vi "Actor Core.vi"(8 "error in":errorcluster, 11 "Main in":refnum<class "Main.lvclass">) -> (0 "error out":errorcluster, 3 "Actor out":refnum<class "Actor.lvclass">)   [LabVIEW 2023, in "Main.lvlib" / "Main.lvclass"]
doc: "The user interface for this panel.\n\n----\nPlease see the following web address for additional documentation and tutorial information:\nhttp://www.mooregoodideas.com/mgi-panel-manager/\n\nAuthor: Derek Trepanier\n\nCopyright (c) 2018, Moore Good Ideas, Inc.\n\nAll rights reserved.\n\nRedistribution and use in source and binary forms, with or without modification, are permitted provided that the following conditions are met:\n\n * Redistributions of source code must retain the above copyright notice, this list of conditions and the following disclaimer.\n * Redistributions in binary form must reproduce the above copyright notice, this list of conditions and the following disclaimer in the documentation and/or other materials provided with the distribution.\n * Neither the name of Moore Good Ideas, Inc. nor the names of its contributors may be used to endorse or promote products derived from this software without specific prior written permission.\n\nTHIS SOFTWARE IS PROVIDED BY THE COPYRIGHT HOLDERS AND CONTRIBUTORS \"AS IS\" AND ANY EXPRESS OR IMPLIED WARRANTIES, INCLUDING, BUT NOT LIMITED TO, THE IMPLIED WARRANTIES OF MERCHANTABILITY AND FITNESS FOR A PARTICULAR PURPOSE ARE DISCLAIMED. IN NO EVENT SHALL THE COPYRIGHT OWNER OR CONTRIBUTORS BE LIABLE FOR ANY DIRECT, INDIRECT, INCIDENTAL, SPECIAL, EXEMPLARY, OR CONSEQUENTIAL DAMAGES (INCLUDING, BUT NOT LIMITED TO, PROCUREMENT OF SUBSTITUTE GOODS OR SERVICES; LOSS OF USE, DATA, OR PROFITS; OR BUSINESS INTERRUPTION) HOWEVER CAUSED AND ON ANY THEORY OF LIABILITY, WHETHER IN CONTRACT, STRICT LIABILITY, OR TORT (INCLUDING NEGLIGENCE OR OTHERWISE) ARISING IN ANY WAY OUT OF THE USE OF THIS SOFTWARE, EVEN IF ADVISED OF THE POSSIBILITY OF SUCH DAMAGE."
uses:
  Library/Main.lvclass
  builds/Framework/Actor Framework.lvlibp/1abvi3w/vi.lib/ActorFramework/Actor/Actor.lvclass
  Main Messages/Menu Response Msg/Menu Response Msg.lvclass/Menu Response Msg.ctl
  builds/Framework/Actor Framework.lvlibp/1abvi3w/vi.lib/ActorFramework/Message Enqueuer/Enqueue.vi
  Main Messages/Menu Response Msg/Menu Response Msg.lvclass
  builds/Framework/Engine.lvlibp/Managed Actor/Library/Managed Actor.lvclass
  builds/Framework/Engine.lvlibp/Engine/Library/Engine.lvclass
  builds/Framework/Actor Framework.lvlibp/1abvi3w/vi.lib/ActorFramework/Stop Msg/Stop Msg.lvclass
  C:/Users/Public/Documents/Development/builds/Framework/Engine.lvlibp/Engine/Library/Engine.lvclass
panel:
  in  "report":bool
  in  "configuration":bool
  in  "manual":bool
  in  "login":bool
  in  "uutinfo":bool
  out "Up Time:":string
  out "Serial:":string
  out "Model:":string
  out "Witness:":string
  out "Operator:":string
  out "Status":string
  out "Version":string caption="v"
  out "MissionLogo":picture
  out "CompanyLogo":picture
  out "Time":timestamp format="%<%I:%M:%S %p\n%x>T"
  in  "E-Stop":bool
  out "SplashScreen":picture
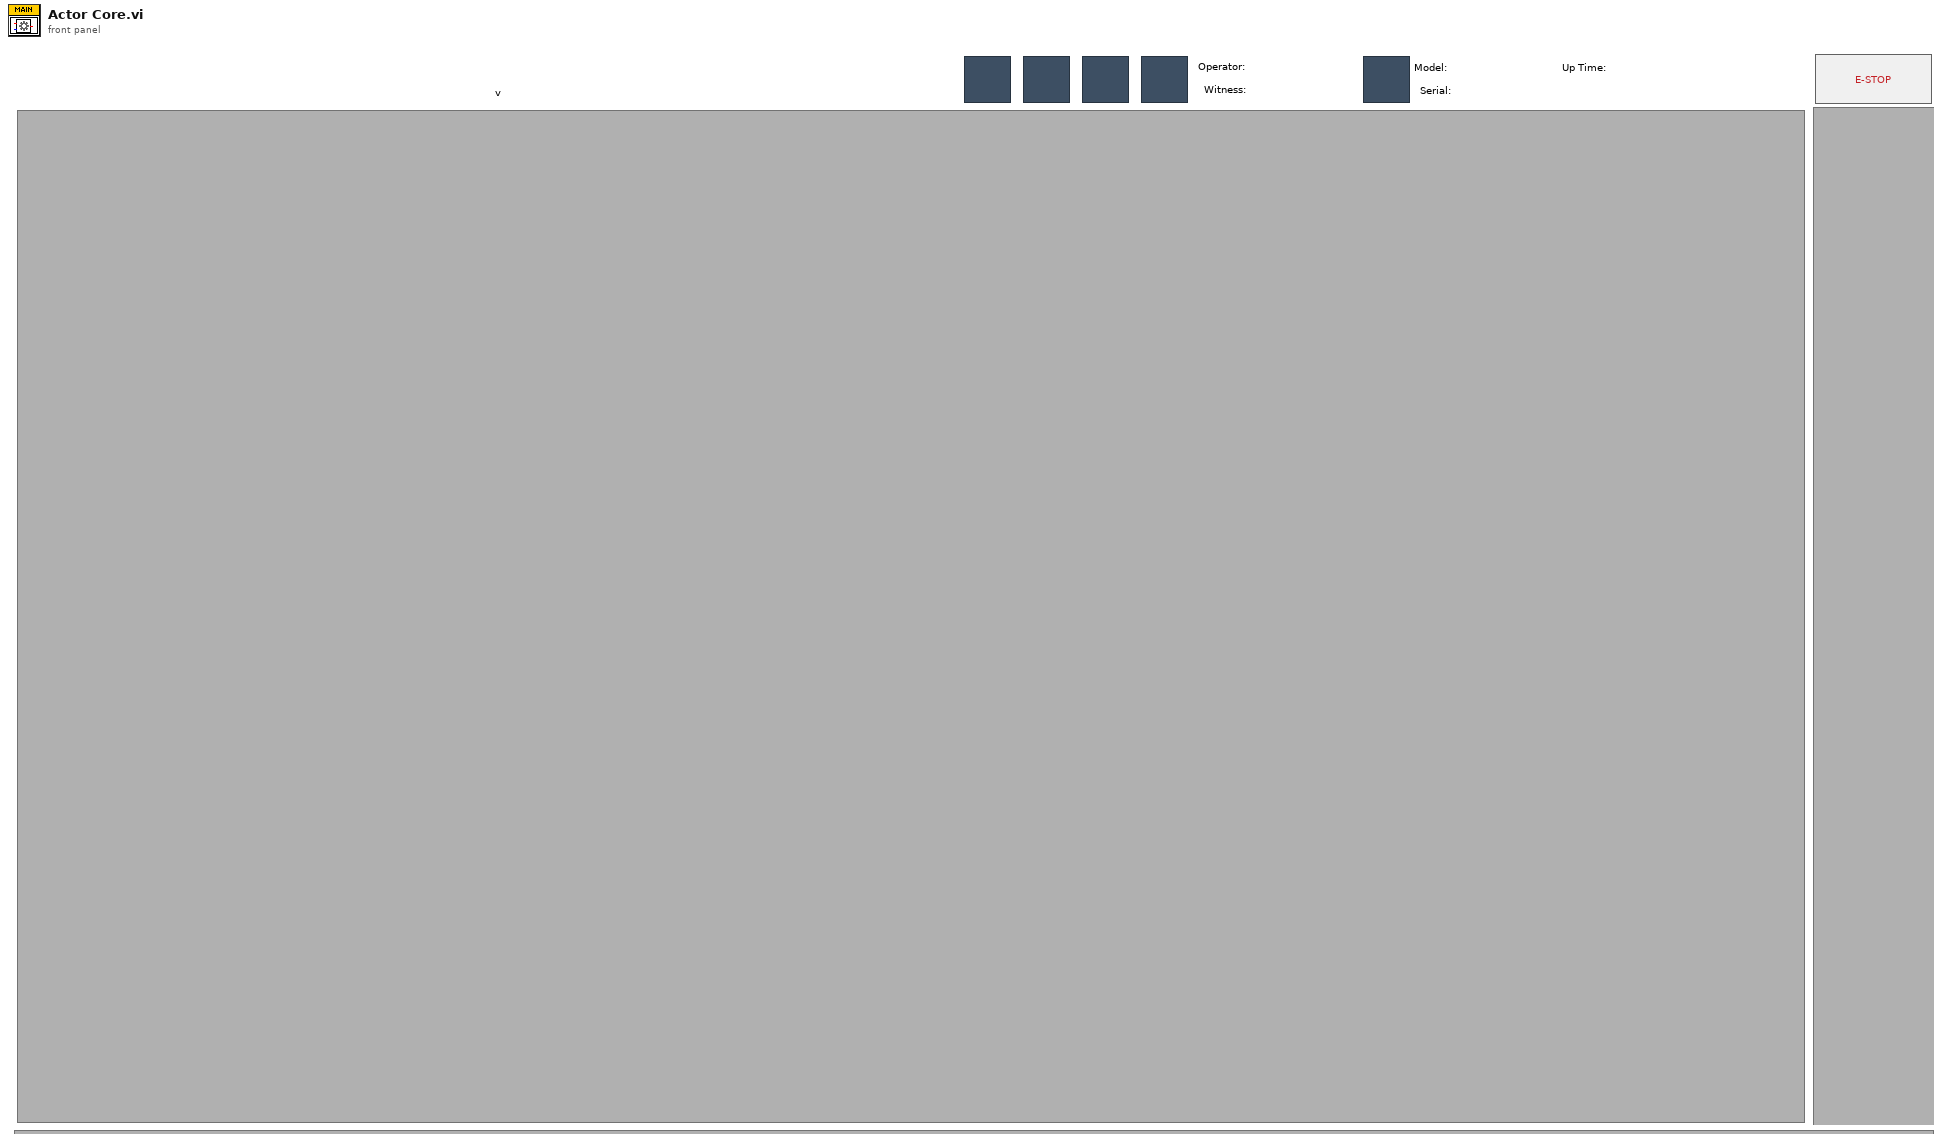
[diagram p1: front panel]
types:
  T1 = cluster{"Pnl Actor":refnum<event-registration>, "Event Registration Refnum":refnum<event-registration>}
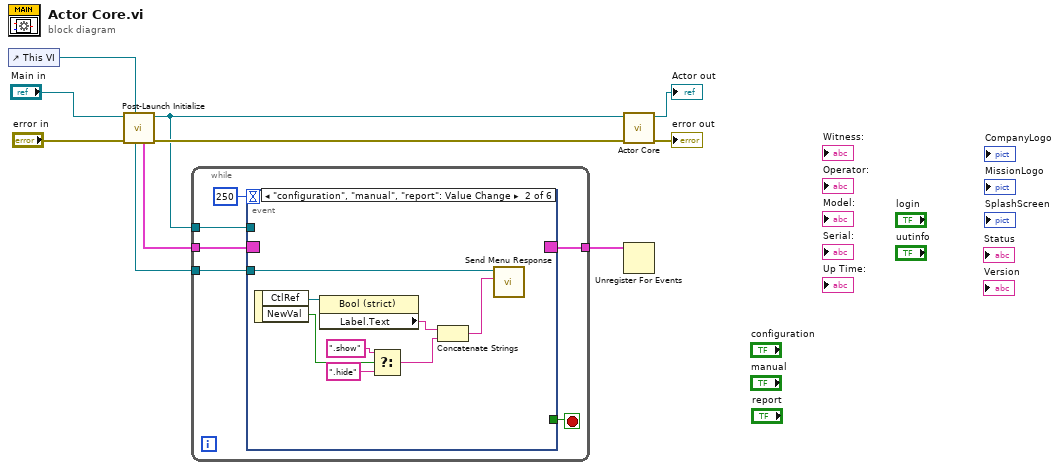
[diagram p0: block diagram]
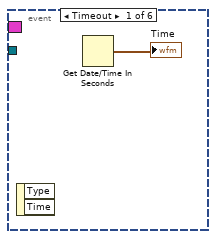
[diagram p2: hidden frame]
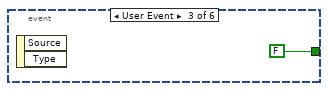
[diagram p3: hidden frame]
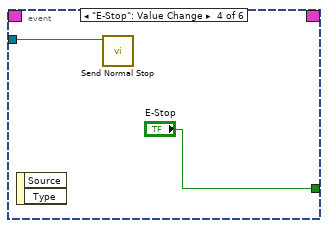
[diagram p4: hidden frame]
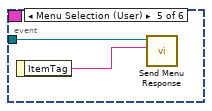
[diagram p5: hidden frame]
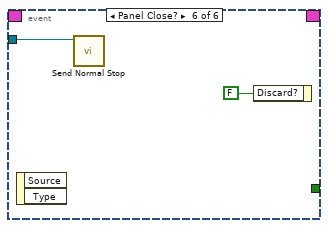
[diagram p6: hidden frame]
diagram:
  n1 = control-ref of="This VI"() -> (w5:refnum<vi>)
  n2 = call "Post-Launch Initialize.vi"("GUI Reference"=w5, "error in (no error)"="error in", "Engine in"="Main in") -> ("error out"=w7:errorcluster, "Engine out"=w3:refnum<class "Main.lvclass">, "Registered Events"=w4:T1, "Self Enqueuer"=w2:refnum<class "Message Enqueuer.lvclass">)  [unwired: 5 in]
  n3 = while {
    tunnel: w4 -> [w16]
    tunnel: w3 -> [w15]
    tunnel: w2 -> [w14]
    tunnel: [w12] -> w1
    stop <- w13 stop-if-true
    n4 = event shown="[1] \"configuration\", \"manual\", \"report\": Value Change" {
      selector: w16 -> [_ _ _ _ _ _]
      dyn-events: [_ _ _ _ _ _] -> w12
      timeout: 250 -> [_ _ _ _ _ _]
      tunnel: w15 -> [_ _ _ _ _ _]
      tunnel: w14 -> [_ w19 _ w28 w30 w31]
      tunnel: [_ _ FALSE "E-Stop" _ _] -> w13
      event Timeout {
        n5 = event-data() -> ()  [unwired: 1 in, 2 out]
        n6 = Get Date/Time In Seconds() -> (seconds since 1Jan1904=→"Time":timestamp)
      }
      event "configuration", "manual", "report": Value Change {
        n7 = event-data() -> ("CtlRef"=w25:refnum<vi>, "NewVal"=w22:bool)  [unwired: 1 in]
        n8 = property class="Bool (strict)"(reference=w25) -> ("Label.Text"=w21:string)  [unwired: 1 in, 2 out]
        n9 = Select(t=".show", s=w22, f=".hide") -> (s? t:f=w20:string)
        n10 = Concatenate Strings(w21, w20) -> (w18:string)
        n11 = call "Send Menu Response.vi"("Menu Tag"=w18, "Message Enqueuer"=w19) -> ()  [unwired: 8 in, 2 out]
      }
      event User Event {
        n12 = event-data() -> ()  [unwired: 1 in, 2 out]
      }
      event "E-Stop": Value Change {
        n13 = event-data() -> ()  [unwired: 1 in, 2 out]
        n14 = call "Send Normal Stop.vi"("Message Enqueuer"=w28) -> ()  [unwired: 10 in, 1 out]
      }
      event Menu Selection (User) {
        n15 = event-data() -> ("ItemTag"=w29:string)  [unwired: 1 in]
        n16 = call "Send Menu Response.vi"("Menu Tag"=w29, "Message Enqueuer"=w30) -> ()  [unwired: 8 in, 2 out]
      }
      event Panel Close? {
        n17 = event-data() -> ()  [unwired: 1 in, 2 out]
        n18 = call "Send Normal Stop.vi"("Message Enqueuer"=w31) -> ()  [unwired: 10 in, 1 out]
        n19 = event-data("Discard?"=FALSE) -> ()  [unwired: 1 in, 1 out]
      }
    }
  }
  n20 = call-parent "Actor Core.vi"("error in"=w7, "Panel Actor in"=w3) -> ("error out"=→"error out":errorcluster, "Actor out"=→"Actor out":refnum<class "Actor.lvclass">)  [unwired: 8 in]
  n21 = Unregister For Events(event registration refnum=w1) -> ()  [unwired: 1 in, 1 out]
